vi "4.register-while-previous-loop-view.vi"() -> ()   [LabVIEW 2016]
panel:
  out "previous":dbl
  out "x+y =":i32
  out "Iteration-no":dbl
  in  "stop":bool
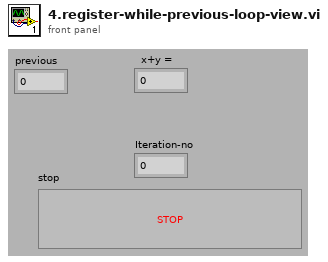
[diagram p1: front panel]
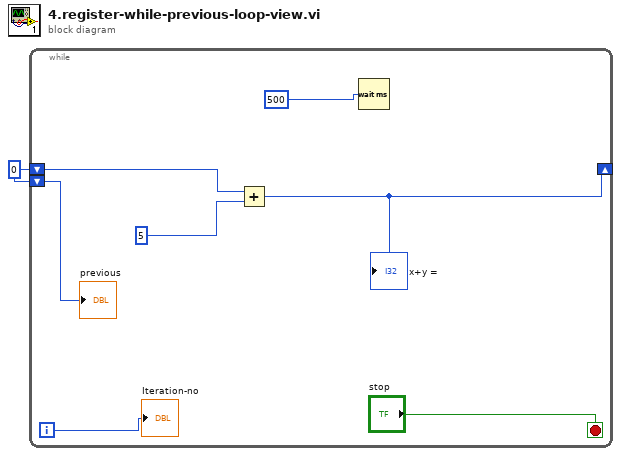
[diagram p0: block diagram]
diagram:
  w1 = 0
  n1 = while {
    shift-right: [w4] -> _
    shift-left: w1 -> [w5]
    shift-left: w1 -> [w2]
    i -> [w7]
    stop <- "stop" stop-if-true
    n2 = Add(x=w5, y=5) -> (x+y=w4:i32)
    "x+y =" <- w4
    n3 = Wait (ms)(milliseconds to wait=500) -> ()  [unwired: 1 out]
    "Iteration-no" <- w7
    "previous" <- w2
  }
